vi "Set All Filters.vi"(8 "error in (no error)":errorcluster, 10 "Filter Wheel Position":i32[](array[numeric]), 11 "FW Arduino Control in":refnum<class "FW Arduino Control.lvclass">) -> (0 "error out":errorcluster, 3 "FW Arduino Control out":refnum<class "FW Arduino Control.lvclass">)   [LabVIEW 2024, in "FW Arduino Control.lvclass"]
uses:
  FW Arduino Control.lvclass
  C:/Development/Prime-RIMAS/Filter Wheel/Filter Wheel Object/Filter Wheel.lvclass
  FW Arduino Control.lvclass/FW Arduino Control.ctl
  Filter Wheel Object/Filter Wheel.lvclass
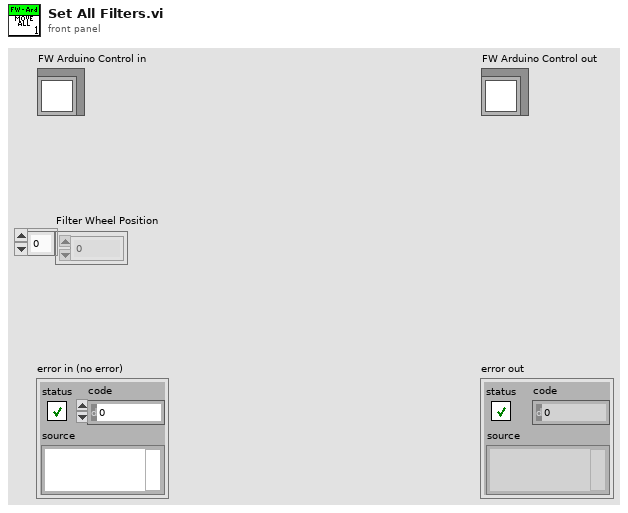
[diagram p1: front panel]
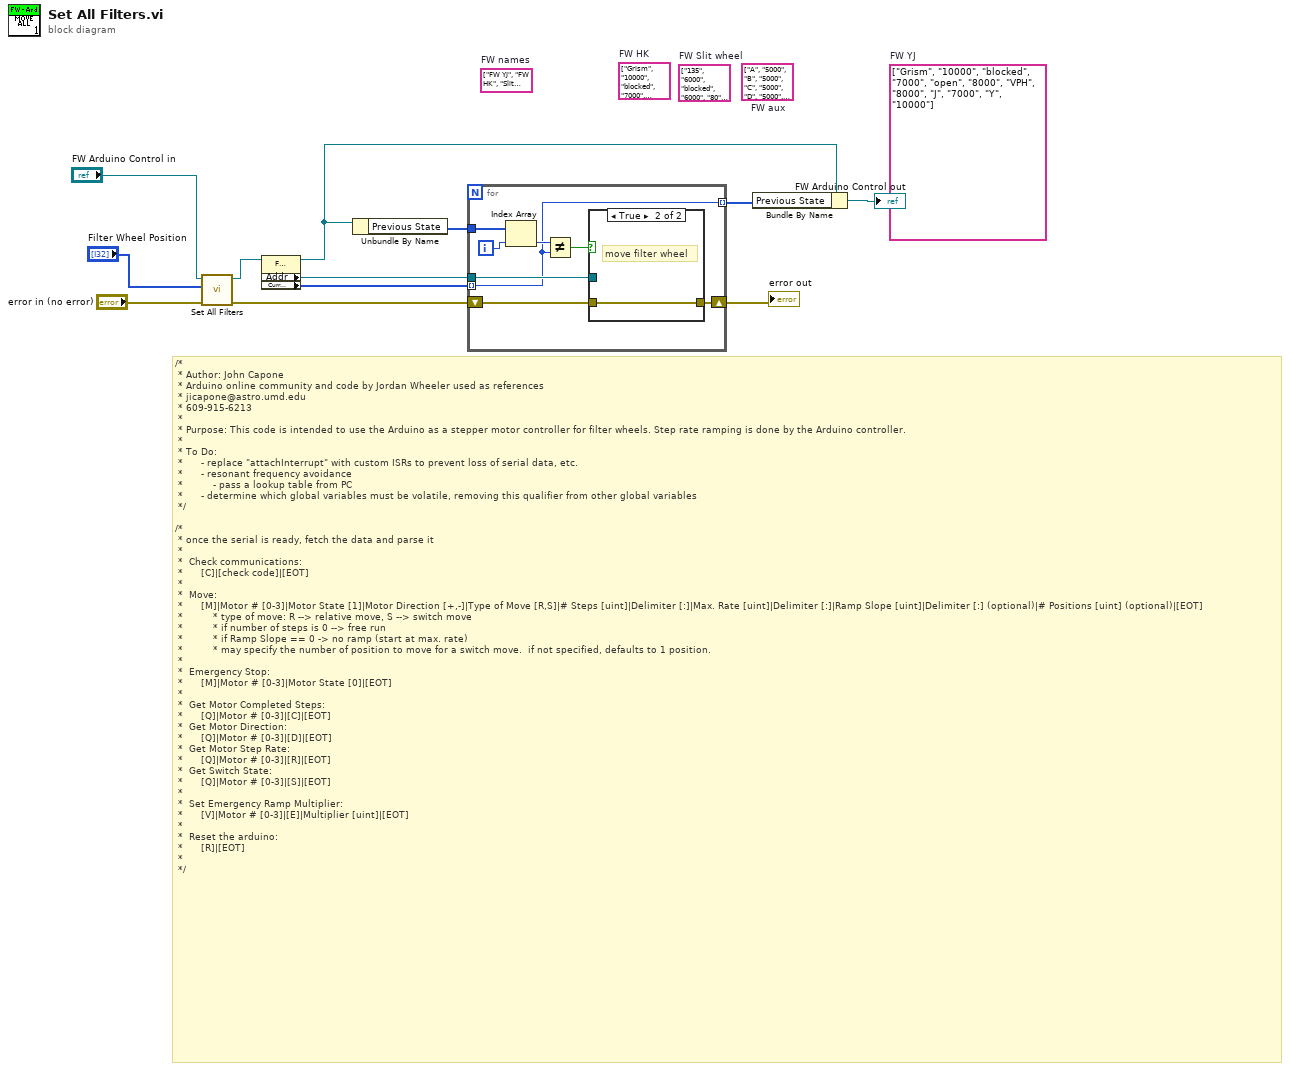
[diagram p0: block diagram]
diagram:
  (unwired) string[] ["FW YJ", "FW HK", "Slit wheel", "FW aux"]  # FW names
  (unwired) string[][] [["Grism", "10000"], ["blocked", "7000"], ["open", "8000"], ["VPH", "8000"], ["J", "7000"], ["Y", "10000"]]  # FW YJ
  (unwired) string[][] [["Grism", "10000"], ["blocked", "7000"], ["open", "8000"], ["VPH", "8000"], ["H", "7000"], ["K", "10000"]]  # FW HK
  (unwired) string[][] [["135", "6000"], ["blocked", "6000"], ["80", "7000"], ["open 1", "7000"], ["250", "7000"], ["open", "7000"]]  # FW Slit wheel
  (unwired) string[][] [["A", "5000"], ["B", "5000"], ["C", "5000"], ["D", "5000"], ["E", "5000"], ["F", "5000"], ["G", "5000"], ["H", "5000"]]  # FW aux
  # "/*\n * Author: John Capone\n * Arduino online community and code by Jordan Wheeler used as references\n * jicapone@astro.umd.edu\n * 609-915-6213\n * \n * Purpose: This code is intended to use the Arduino as a stepper motor controller for filter wheels. Step rate ramping is done by the Arduino controller.\n * \n * To Do:\n *      - replace \"attachInterrupt\" with custom ISRs to prevent loss of serial data, etc.\n *      - resonant frequency avoidance\n *          - pass a lookup table from PC\n *      - determine which global variables must be volatile, removing this qualifier from other global variables\n */\n\n/* \n * once the serial is ready, fetch the data and parse it\n *\n *  Check communications:\n *      [C]|[check code]|[EOT]\n *\n *  Move:\n *      [M]|Motor # [0-3]|Motor State [1]|Motor Direction [+,-]|Type of Move [R,S]|# Steps [uint]|Delimiter [:]|Max. Rate [uint]|Delimiter [:]|Ramp Slope [uint]|Delimiter [:] (optional)|# Positions [uint] (optional)|[EOT]\n *          * type of move: R --> relative move, S --> switch move\n *          * if number of steps is 0 --> free run\n *          * if Ramp Slope == 0 -> no ramp (start at max. rate)\n *          * may specify the number of position to move for a switch move.  if not specified, defaults to 1 position.\n *\n *  Emergency Stop:\n *      [M]|Motor # [0-3]|Motor State [0]|[EOT]\n *\n *  Get Motor Completed Steps:\n *      [Q]|Motor # [0-3]|[C]|[EOT]\n *  Get Motor Direction:\n *      [Q]|Motor # [0-3]|[D]|[EOT]\n *  Get Motor Step Rate:\n *      [Q]|Motor # [0-3]|[R]|[EOT]\n *  Get Switch State:\n *      [Q]|Motor # [0-3]|[S]|[EOT]\n *\n *  Set Emergency Ramp Multiplier:\n *      [V]|Motor # [0-3]|[E]|Multiplier [uint]|[EOT]\n *\n *  Reset the arduino:\n *      [R]|[EOT]\n *\n */"
  n1 = call-parent "Set All Filters.vi"("error in (no error)"="error in (no error)", "Filter Wheel Position"="Filter Wheel Position", "Filter Wheel in"="FW Arduino Control in") -> ("error out"=w10:errorcluster, "Filter Wheel out"=w5:refnum<class "FW Arduino Control.lvclass">)  [unwired: 7 in]
  n2 = property class="FW Arduino Control.lvclass"(reference=w5) -> (reference out=w4:refnum<class "FW Arduino Control.lvclass">, "Addr"=w3:refnum<visa-resource-name>, "Curr Position"=w2:i32[])  [unwired: 1 in, 1 out]
  n3 = Unbundle By Name(w4) -> ("Previous State"=w9:i32[])
  n4 = for {
    tunnel: w2 -> [w13] mode=indexing
    tunnel: w3 -> [w16]
    tunnel: w9 -> [w20]
    shift-right: [w14] -> w6
    shift-left: w10 -> [w15]
    tunnel: [w13] -> w8 mode=indexing
    i -> [w19]
    n5 = Index Array(array=w20, index=w19) -> (element=w18:i32)
    n6 = Not Equal?(x=w18, y=w13) -> (x != y?=w17:bool)
    n7 = case shown="True" w17 {
      tunnel: w16 -> [_ _]
      tunnel: w15 -> [w21 w22]
      tunnel: [w21 w22] -> w14
      frame False {
        # "already in \nposition"
      }
      frame True {
        # "move filter wheel"
      }
    }
  }
  "error out" <- w6
  n8 = Bundle By Name(cluster=w4, "Previous State"=w8) -> (→"FW Arduino Control out":refnum<class "FW Arduino Control.lvclass">)
